vi "Interpret Driver Controls.vi"   [LabVIEW 2018]
uses:
  SubSystems/Controllers/Driver Controller/Driver Controller Global.vi
  SubSystems/Drive Train/Drive Train Global.vi
  SubSystems/Lift/Lift Global.vi
  SubSystems/Controllers/Manipulator Controlller/Manipulator Controller Global.vi
  SubSystems/Cargo Intake/Cargo Intake Global.vi
  SubSystems/HAB Climber/HAB Climber Global.vi
  SubSystems/Hatch Panel Intake/Hatch Panel Intake Global.vi
types:
  T1 = cluster{"Rollover":dbl, "Yaw":dbl, "Cont Yaw":dbl}
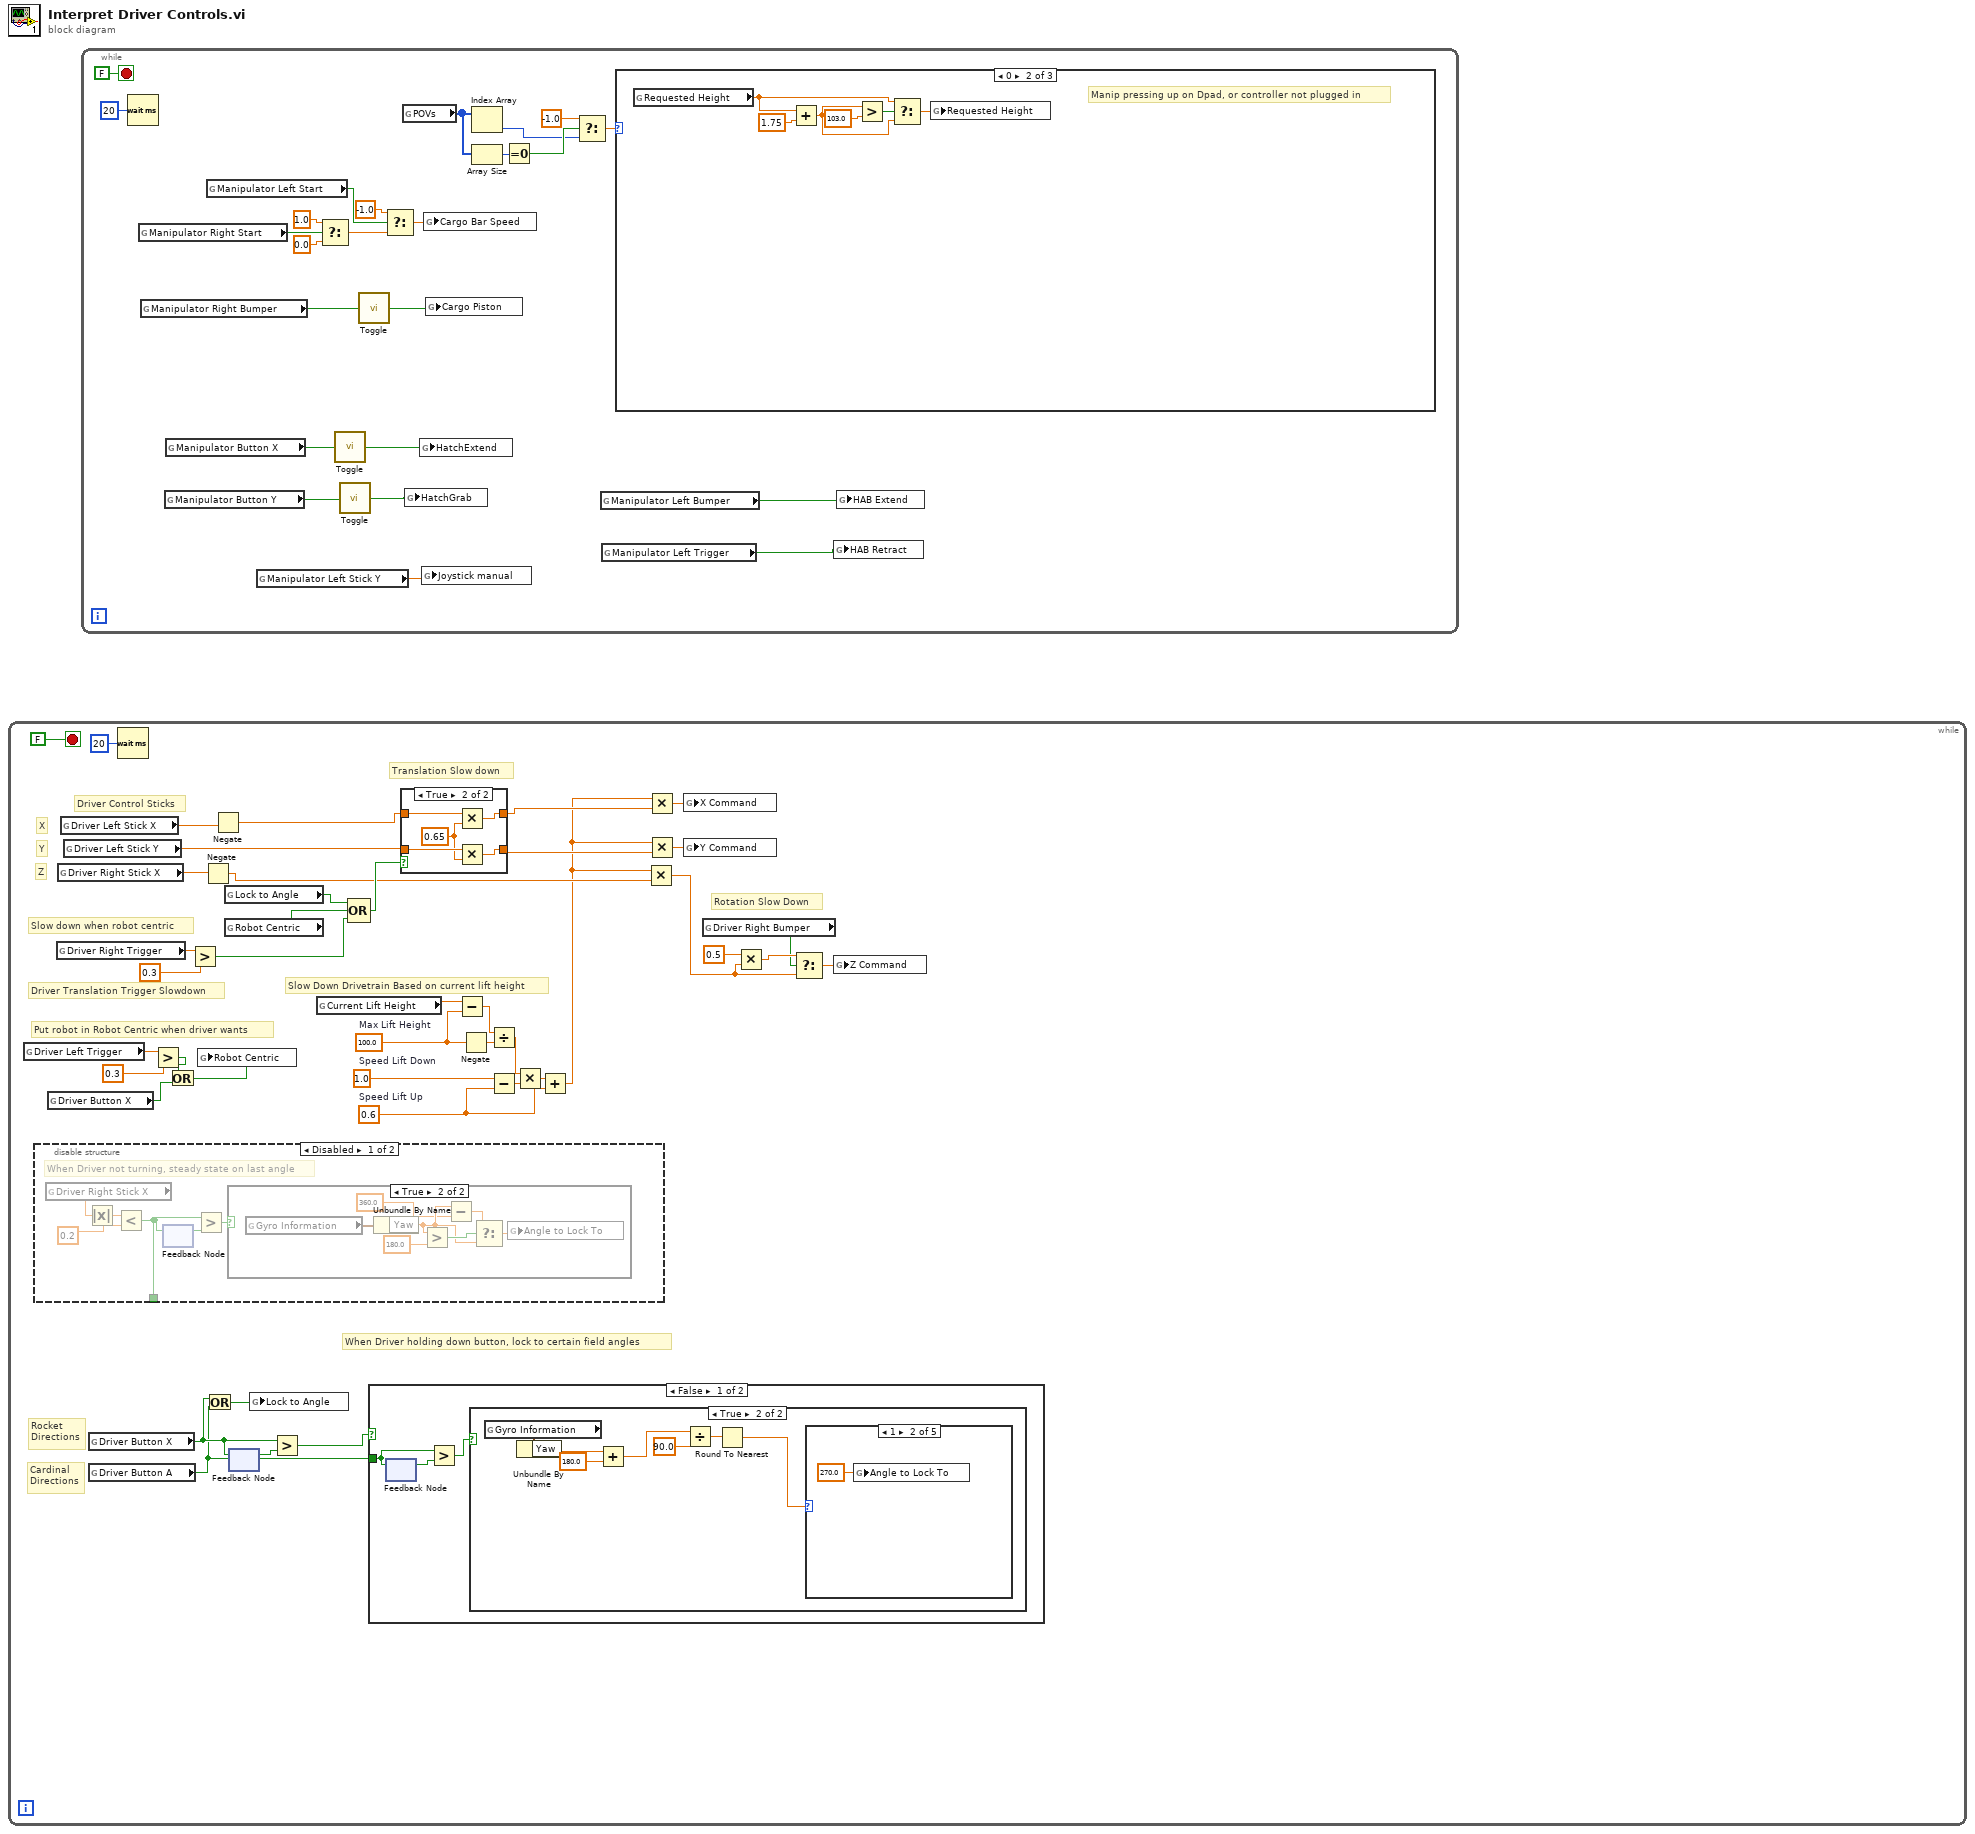
[diagram p0: block diagram]
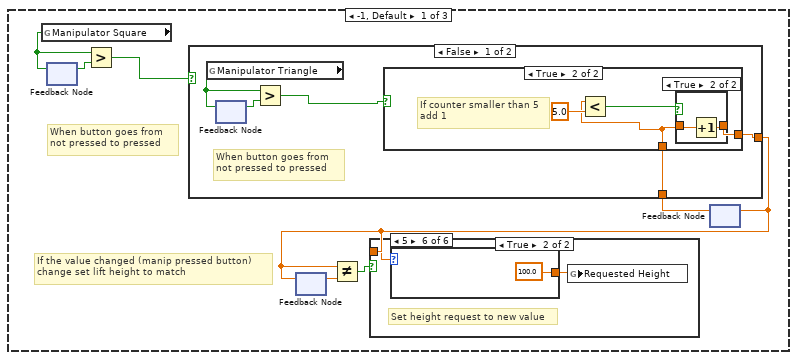
[diagram p2: hidden frame]
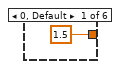
[diagram p4: hidden frame]
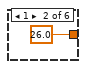
[diagram p5: hidden frame]
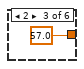
[diagram p6: hidden frame]
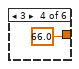
[diagram p7: hidden frame]
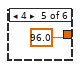
[diagram p8: hidden frame]
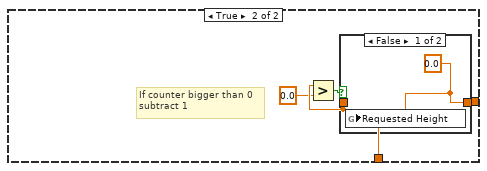
[diagram p11: hidden frame]
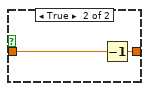
[diagram p12: hidden frame]
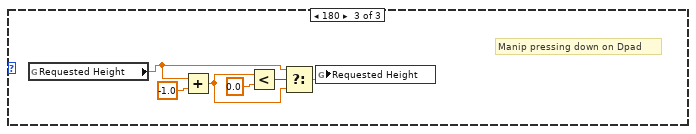
[diagram p13: hidden frame]
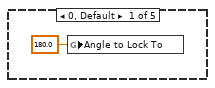
[diagram p17: hidden frame]
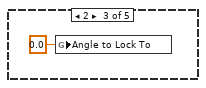
[diagram p18: hidden frame]
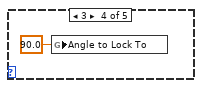
[diagram p19: hidden frame]
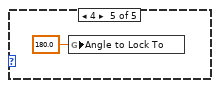
[diagram p20: hidden frame]
diagram:
  n1 = while {
    stop <- FALSE stop-if-true
    w13 = 0.6  # Speed Lift Up
    w17 = 1.0  # Speed Lift Down
    w11 = 100.0  # Max Lift Height
    # "Rotation Slow Down"
    # "Rocket\nDirections"
    # "Cardinal\nDirections"
    # "When Driver holding down button, lock to certain field angles"
    # "Slow Down Drivetrain Based on current lift height"
    # "Put robot in Robot Centric when driver wants"
    # "Slow down when robot centric"
    # "Driver Translation Trigger Slowdown"
    # "Translation Slow down"
    # "Z"
    # "Y"
    # "X"
    # "Driver Control Sticks"
    n2 = global read "Driver Controller Global.vi" "Driver Left Trigger"() -> (w33:dbl)
    n3 = disable-structure shown="Disabled" {
      disable-tunnel: [w43 _] -> _
      frame Disabled {
        # "When Driver not turning, steady state on last angle"
        n4 = global read "Driver Controller Global.vi" "Driver Right Stick X"() -> (w44:dbl)
        n5 = Absolute Value(x=w44) -> (abs(x)=w48:dbl)
        n6 = Less?(x=w48, y=0.2) -> (x < y?=w43:bool)
        n7 = feedback #1() -> (w46:bool)  [unwired: 1 in]
        n8 = feedback-in #1(w43) -> ()
        n9 = Greater?(x=w43, y=w46) -> (0:w45:bool)
        n10 = case shown="True" w45 {
          frame False {
          }
          frame True {
            n11 = global read "Drive Train Global.vi" "Gyro Information"() -> (w55:T1)
            n12 = Unbundle By Name(w55) -> ("Yaw"=w52:dbl)
            n13 = Greater?(x=w52, y=180.0) -> (0:w53:bool)
            n14 = Subtract(x=w52, y=360.0) -> (x-y=w50:dbl)
            n15 = Select(t=w50, s=w53, f=w52) -> (s? t:f=w49:dbl)
            n16 = global write "Drive Train Global.vi" "Angle to Lock To"(w49) -> ()
          }
        }
      }
      frame Enabled {
      }
    }
    n17 = global read "Driver Controller Global.vi" "Driver Button X"() -> (w2:bool)
    n18 = global read "Driver Controller Global.vi" "Driver Right Trigger"() -> (w38:dbl)
    n19 = global read "Driver Controller Global.vi" "Driver Right Stick X"() -> (w39:dbl)
    n20 = global read "Driver Controller Global.vi" "Driver Left Stick X"() -> (w40:dbl)
    n21 = global read "Driver Controller Global.vi" "Driver Left Stick Y"() -> (w20:dbl)
    n22 = global read "Driver Controller Global.vi" "Driver Button X"() -> (w8:bool)
    n23 = global read "Driver Controller Global.vi" "Driver Button A"() -> (w6:bool)
    n24 = Wait (ms)(milliseconds to wait=u32 20) -> ()  [unwired: 1 out]
    n25 = Greater?(x=w33, y=0.3) -> (0:w4:bool)
    n26 = Or(x=w4, y=w2) -> (x .or. y?=w3:bool)
    n27 = Greater?(x=w38, y=0.3) -> (0:w28:bool)
    n28 = global write "Drive Train Global.vi" "Robot Centric"(w3) -> ()
    n29 = Negate(x=w39) -> (-x=w24:dbl)
    n30 = Or(x=w8, y=w6) -> (x .or. y?=w5:bool)
    n31 = Negate(x=w40) -> (-x=w21:dbl)
    n32 = global read "Drive Train Global.vi" "Lock to Angle"() -> (w1:bool)
    n33 = global read "Drive Train Global.vi" "Robot Centric"() -> (w27:bool)
    n34 = feedback #2() -> (w9:bool)  [unwired: 1 in]
    n35 = feedback-in #2(w8) -> ()
    n36 = global write "Drive Train Global.vi" "Lock to Angle"(w5) -> ()
    n37 = Greater?(x=w8, y=w9) -> (0:w7:bool)
    n38 = global read "Lift Global.vi" "Current Lift Height"() -> (w19:dbl)
    n39 = Compound Arithmetic op=OR(w1, w27, w28) -> (w26:bool)
    n40 = case shown="False" w7 {
      tunnel: w6 -> [w57 _]
      frame False {
        n41 = feedback #3() -> (w58:bool)  [unwired: 1 in]
        n42 = feedback-in #3(w57) -> ()
        n43 = Greater?(x=w57, y=w58) -> (0:w56:bool)
        n44 = case shown="True" w56 {
          frame False {
          }
          frame True {
            n45 = global read "Drive Train Global.vi" "Gyro Information"() -> (w65:T1)
            n46 = Unbundle By Name(w65) -> ("Yaw"=w62:dbl)
            n47 = Add(x=w62, y=180.0) -> (x+y=w61:dbl)
            n48 = Divide(x=w61, y=90.0) -> (x/y=w63:dbl)
            n49 = Round To Nearest(number=w63) -> (nearest integer value=w59:dbl)
            n50 = case shown="1" w59 {
              frame 0, Default {
                n51 = global write "Drive Train Global.vi" "Angle to Lock To"(180.0 ("Angle to Lock To")) -> ()
              }
              frame 1 {
                n52 = global write "Drive Train Global.vi" "Angle to Lock To"(270.0 ("Angle to Lock To")) -> ()
              }
              frame 2 {
                n53 = global write "Drive Train Global.vi" "Angle to Lock To"(0.0 ("Angle to Lock To")) -> ()
              }
              frame 3 {
                n54 = global write "Drive Train Global.vi" "Angle to Lock To"(90.0 ("Angle to Lock To")) -> ()
              }
              frame 4 {
                n55 = global write "Drive Train Global.vi" "Angle to Lock To"(180.0 ("Angle to Lock To")) -> ()
              }
            }
          }
        }
      }
      frame True {
        n56 = global read "Drive Train Global.vi" "Gyro Information"() -> (w79:T1)
        n57 = Unbundle By Name(w79) -> ("Cont Yaw"=w77:dbl)
        n58 = Quotient & Remainder(x=w77, y=360.0) -> (x-y*floor(x/y)=w75:dbl)  [unwired: 1 out]
        n59 = Divide(x=w75, y=60.0) -> (x/y=w71:dbl)
        n60 = In Range and Coerce(upper limit=1.5, x=w71, lower limit=0.0) -> (In Range?=w72:bool)  [unwired: 1 out]
        n61 = case shown="False" w72 {
          tunnel: w71 -> [w80 _]
          frame False {
            n62 = In Range and Coerce(upper limit=3.0, x=w80, lower limit=1.5) -> (In Range?=w81:bool)  [unwired: 1 out]
            n63 = case shown="False" w81 {
              tunnel: w80 -> [w86 _]
              tunnel: w80 -> [w84 _]
              frame False {
                n64 = In Range and Coerce(upper limit=4.5, x=w86, lower limit=3.0) -> (In Range?=w85:bool)  [unwired: 1 out]
                n65 = case shown="False" w85 {
                  tunnel: w84 -> [w90 _]
                  frame False {
                    n66 = In Range and Coerce(upper limit=6.0, x=w90, lower limit=4.5) -> (In Range?=w89:bool)  [unwired: 1 out]
                    n67 = case shown="True" w89 {
                      frame False {
                      }
                      frame True {
                        n68 = global write "Drive Train Global.vi" "Angle to Lock To"(330.0 ("Angle to Lock To")) -> ()
                      }
                    }
                  }
                  frame True {
                    n69 = global write "Drive Train Global.vi" "Angle to Lock To"(210.0 ("Angle to Lock To")) -> ()
                  }
                }
              }
              frame True {
                n70 = global write "Drive Train Global.vi" "Angle to Lock To"(150.0 ("Angle to Lock To")) -> ()
              }
            }
          }
          frame True {
            n71 = global write "Drive Train Global.vi" "Angle to Lock To"(30.0 ("Angle to Lock To")) -> ()
          }
        }
      }
    }
    n72 = case shown="True" w26 {
      tunnel: w20 -> [w98 w103]
      tunnel: [w98 w102] -> w23
      tunnel: [w97 w101] -> w22
      tunnel: w21 -> [w97 w100]
      frame False {
      }
      frame True {
        w99 = 0.65 ("Y Slower")
        n73 = Multiply(x=w100, y=w99) -> (x*y=w101:dbl)
        n74 = Multiply(x=w103, y=w99) -> (x*y=w102:dbl)
      }
    }
    n75 = Subtract(x=w19, y=w11) -> (x-y=w18:dbl)
    n76 = Negate(x=w11) -> (-x=w12:dbl)
    n77 = Divide(x=w18, y=w12) -> (x/y=w16:dbl)
    n78 = Subtract(x=w17, y=w13) -> (x-y=w15:dbl)
    n79 = Multiply(x=w16, y=w15) -> (x*y=w14:dbl)
    n80 = Add(x=w14, y=w13) -> (x+y=w10:dbl)
    n81 = Multiply(x=w10, y=w24) -> (x*y=w32:dbl)
    n82 = Multiply(x=w10, y=w22) -> (x*y=w36:dbl)
    n83 = Multiply(x=w10, y=w23) -> (x*y=w35:dbl)
    n84 = global write "Drive Train Global.vi" "X Command"(w36) -> ()
    n85 = global write "Drive Train Global.vi" "Y Command"(w35) -> ()
    n86 = global read "Driver Controller Global.vi" "Driver Right Bumper"() -> (w29:bool)
    n87 = Multiply(x=0.5, y=w32) -> (x*y=w31:dbl)
    n88 = Select(t=w31, s=w29, f=w32) -> (s? t:f=w25:dbl)
    n89 = global write "Drive Train Global.vi" "Z Command"(w25) -> ()
  }
  n90 = while {
    stop <- FALSE stop-if-true
    n91 = Wait (ms)(milliseconds to wait=u32 20) -> ()  [unwired: 1 out]
    n92 = global read "Manipulator Controller Global.vi" "Manipulator Right Start"() -> (w122:bool)
    n93 = global read "Manipulator Controller Global.vi" "Manipulator Right Bumper"() -> (w125:bool)
    n94 = global read "Manipulator Controller Global.vi" "Manipulator Button Y"() -> (w116:bool)
    n95 = global read "Manipulator Controller Global.vi" "Manipulator Button X"() -> (w114:bool)
    n96 = global read "Manipulator Controller Global.vi" "Manipulator Left Start"() -> (w121:bool)
    n97 = global read "Manipulator Controller Global.vi" "Manipulator Left Stick Y"() -> (w106:dbl)
    n98 = Select(t=1.0, s=w122, f=0.0) -> (s? t:f=w120:dbl)
    n99 = call "Toggle.vi"("Input"=w114) -> ("Output"=w115:bool)
    n100 = call "Toggle.vi"("Input"=w116) -> ("Output"=w107:bool)
    n101 = call "Toggle.vi"("Input"=w125) -> ("Output"=w124:bool)
    n102 = Select(t=-1.0, s=w121, f=w120) -> (s? t:f=w123:dbl)
    n103 = global read "Manipulator Controller Global.vi" "POVs"() -> (w113:i16[])
    n104 = global write "Hatch Panel Intake Global.vi" "HatchGrab"(w107) -> ()
    n105 = global write "Hatch Panel Intake Global.vi" "HatchExtend"(w115) -> ()
    n106 = global write "Lift Global.vi" "Joystick manual"(w106) -> ()
    n107 = global write "Cargo Intake Global.vi" "Cargo Bar Speed"(w123) -> ()
    n108 = global write "Cargo Intake Global.vi" "Cargo Piston"(w124) -> ()
    n109 = Index Array(array=w113) -> (element=w108:i16)  [unwired: 1 in]
    n110 = Array Size(array=w113) -> (size(s)=w112:i32)
    n111 = Equal To 0?(x=w112) -> (x = 0?=w110:bool)
    n112 = Select(t=-1.0, s=w110, f=w108) -> (s? t:f=w111:dbl)
    n113 = global read "Manipulator Controller Global.vi" "Manipulator Left Bumper"() -> (w105:bool)
    n114 = global read "Manipulator Controller Global.vi" "Manipulator Left Trigger"() -> (w104:bool)
    n115 = case shown="0" w111 {
      frame -1, Default {
        # "If the value changed (manip pressed button)\nchange set lift height to match"
        # "When button goes from\nnot pressed to pressed"
        n116 = global read "Manipulator Controller Global.vi" "Manipulator Square"() -> (w133:bool)
        n117 = feedback #4() -> (w134:bool)  [unwired: 1 in]
        n118 = feedback-in #4(w133) -> ()
        n119 = Greater?(x=w133, y=w134) -> (0:w128:bool)
        n120 = feedback #5() -> (w131:dbl)  [unwired: 1 in]
        n121 = feedback #6() -> (w132:dbl)  [unwired: 1 in]
        n122 = case shown="False" w128 {
          tunnel: [w144 w159] -> w130
          tunnel: w132 -> [w145 w158]
          frame False {
            # "When button goes from\nnot pressed to pressed"
            n123 = global read "Manipulator Controller Global.vi" "Manipulator Triangle"() -> (w147:bool)
            n124 = feedback #7() -> (w146:bool)  [unwired: 1 in]
            n125 = feedback-in #7(w147) -> ()
            n126 = Greater?(x=w147, y=w146) -> (0:w143:bool)
            n127 = case shown="True" w143 {
              tunnel: w145 -> [w148 w150]
              tunnel: [w148 w152] -> w144
              frame False {
              }
              frame True {
                # "If counter smaller than 5\nadd 1"
                n128 = Less?(x=w150, y=5.0) -> (x < y?=w149:bool)
                n129 = case shown="True" w149 {
                  tunnel: [w153 w155] -> w152
                  tunnel: w150 -> [w153 w154]
                  frame False {
                  }
                  frame True {
                    n130 = Increment(x=w154) -> (x+1=w155:dbl)
                  }
                }
              }
            }
          }
          frame True {
            # "If counter bigger than 0\nsubtract 1"
            n131 = Greater?(x=w158, y=0.0) -> (0:w157:bool)
            n132 = case shown="False" w157 {
              tunnel: [w160 w162] -> w159
              tunnel: w158 -> [_ w161]
              frame False {
                w160 = 0.0 ("y")
                n133 = global write "Lift Global.vi" "Requested Height"(w160) -> ()
              }
              frame True {
                n134 = Decrement(x=w161) -> (x-1=w162:dbl)
              }
            }
          }
        }
        n135 = feedback-in #5(w130) -> ()
        n136 = Not Equal?(x=w130, y=w131) -> (x != y?=w129:bool)
        n137 = case shown="True" w129 {
          tunnel: w130 -> [_ w135]
          frame False {
            # "Manipulator didnt request change"
          }
          frame True {
            # "Set height request to new value"
            n138 = case shown="5" w135 {
              tunnel: [1.5 ("Requested Height") 26.0 ("Requested Height") 57.0 ("Requested Height") 66.0 ("Requested Height") 96.0 ("Requested Height") 100.0 ("Requested Height")] -> w136
              frame 0, Default {
              }
              frame 1 {
              }
              frame 2 {
              }
              frame 3 {
              }
              frame 4 {
              }
              frame 5 {
              }
            }
            n139 = global write "Lift Global.vi" "Requested Height"(w136) -> ()
          }
        }
        n140 = feedback-in #6(w130) -> ()
      }
      frame 0 {
        # "Manip pressing up on Dpad, or controller not plugged in"
        n141 = global read "Lift Global.vi" "Requested Height"() -> (w164:dbl)
        n142 = Add(x=w164, y=1.75) -> (x+y=w163:dbl)
        n143 = Greater?(x=w163, y=103.0) -> (0:w165:bool)
        n144 = Select(t=w164, s=w165, f=w163) -> (s? t:f=w166:dbl)
        n145 = global write "Lift Global.vi" "Requested Height"(w166) -> ()
      }
      frame 180 {
        # "Manip pressing down on Dpad"
        n146 = global read "Lift Global.vi" "Requested Height"() -> (w169:dbl)
        n147 = Add(x=w169, y=-1.0) -> (x+y=w171:dbl)
        n148 = Less?(x=w171, y=0.0) -> (x < y?=w172:bool)
        n149 = Select(t=w169, s=w172, f=w171) -> (s? t:f=w170:dbl)
        n150 = global write "Lift Global.vi" "Requested Height"(w170) -> ()
      }
    }
    n151 = global write "HAB Climber Global.vi" "HAB Retract"(w104) -> ()
    n152 = global write "HAB Climber Global.vi" "HAB Extend"(w105) -> ()
  }
